vi "Set Ramp Rate.vi"(8 "error in (no error)":errorcluster, 11 "Ramp Rate (deg C / second)":dbl) -> (0 "error out":errorcluster)   [LabVIEW 2015, in "Thermal Chamber Response Simulator.lvlib"]
doc: "Set the ramp rate in the simulator AE.\n____\nDelacor QMH Thermal Chamber Examples 4.0.0.21\nCopyright (c) 2018, Delacor"
uses:
  Thermal Chamber Response Simulator.lvlib
  Action--enum.ctl
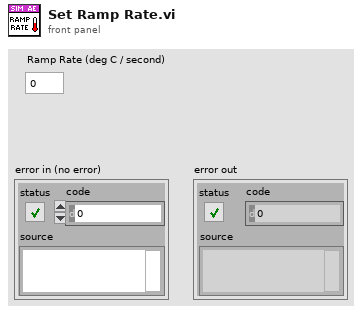
[diagram p1: front panel]
types:
  T1 = typedef "Thermal Chamber Response Simulator.lvlib/Action--enum.ctl" = enum16{"Initialize", "Set Temperature Required", "Set Ramp Rate", "Get Status", "Disable Heater", "Enable Heater", "Exit Application"}
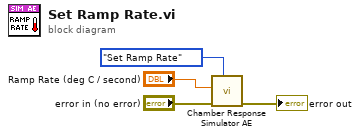
[diagram p0: block diagram]
diagram:
  n1 = call "Chamber Response Simulator AE.vi"("Thermal Chamber Function"=Action--enum."Set Ramp Rate", "error in (no error)"="error in (no error)", "Ramp Rate in"="Ramp Rate (deg C / second)") -> ("error out"=→"error out":errorcluster)  [unwired: 3 in, 5 out]
